vi "ReadImageParameters_JSON(SingleRack).vi"(8 "error in":errorcluster, 9 "Default JSON\nVariant in":variant, 10 "Part Name":string) -> (0 "error out":errorcluster, 2 "Error Message":string, 3 "Cam Enable-Disable Input":T1={"Top Cam"=TRUE, "Side Cam"=FALSE, "Trailing Cam"=FALSE})   [LabVIEW 2015, in "ZenGage v3.0 UI.lvclass"]
uses:
  ZenGage v3.0 UI.lvclass
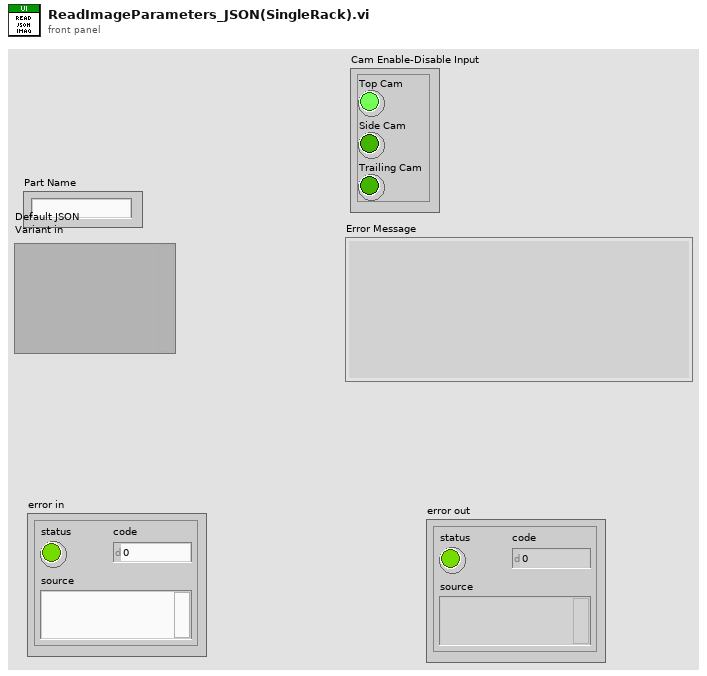
[diagram p1: front panel]
types:
  T1 = cluster{"Top Cam":bool, "Side Cam":bool, "Trailing Cam":bool}
  T2 = cluster{"CameraControllerParameters":cluster{"ID":i32, "NoOfCameras":i32, "CameraID":i32[], "NoOfReceivers":i32, "Diagnostics":cluster{"Path":string, "LightCameraSequence":cluster{"Name":string, "CameraID":i32, "LightID":i32}[], "Delaytime":i32, "DecisionParameters":cluster{"Range":i32[], "AcceptancePercentage":i32[], "Comparison":string[], "AcceptableBlackBinValue":i32}, "DiagnosticsReceiverSequence":cluster{"ReceiverName":string, "ReceiverID":i32}}, "PartsList":cluster{"Name":string, "CameraIDs":i32[], "ReceiverSequence":cluster{"ReceiverName":string, "ReceiverID":i32, "NoOfActiveCameras":i32}[]}[]}[]}
  T3 = cluster{"ID":i32, "NoOfCameras":i32, "CameraID":i32[], "NoOfReceivers":i32, "Diagnostics":cluster{"Path":string, "LightCameraSequence":cluster{"Name":string, "CameraID":i32, "LightID":i32}[], "Delaytime":i32, "DecisionParameters":cluster{"Range":i32[], "AcceptancePercentage":i32[], "Comparison":string[], "AcceptableBlackBinValue":i32}, "DiagnosticsReceiverSequence":cluster{"ReceiverName":string, "ReceiverID":i32}}, "PartsList":cluster{"Name":string, "CameraIDs":i32[], "ReceiverSequence":cluster{"ReceiverName":string, "ReceiverID":i32, "NoOfActiveCameras":i32}[]}[]}[]
  T4 = cluster{"ID":i32, "NoOfCameras":i32, "CameraID":i32[], "NoOfReceivers":i32, "Diagnostics":cluster{"Path":string, "LightCameraSequence":cluster{"Name":string, "CameraID":i32, "LightID":i32}[], "Delaytime":i32, "DecisionParameters":cluster{"Range":i32[], "AcceptancePercentage":i32[], "Comparison":string[], "AcceptableBlackBinValue":i32}, "DiagnosticsReceiverSequence":cluster{"ReceiverName":string, "ReceiverID":i32}}, "PartsList":cluster{"Name":string, "CameraIDs":i32[], "ReceiverSequence":cluster{"ReceiverName":string, "ReceiverID":i32, "NoOfActiveCameras":i32}[]}[]}
  T5 = cluster{"Name":string, "CameraIDs":i32[], "ReceiverSequence":cluster{"ReceiverName":string, "ReceiverID":i32, "NoOfActiveCameras":i32}[]}[]
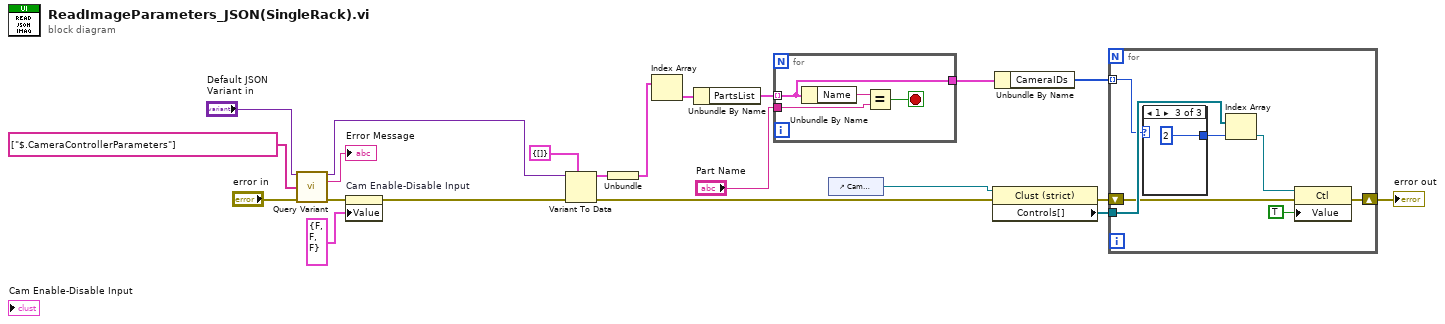
[diagram p0: block diagram]
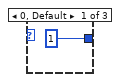
[diagram p2: hidden frame]
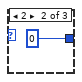
[diagram p3: hidden frame]
diagram:
  n1 = call <vilib>:"Query Variant.vi"("VCluster in"="Default JSON\nVariant in", "pathList"=string[] ["$.CameraControllerParameters"], "error IO"="error in") -> ("VCluster\n out"=w21:variant, "Error Message"=→"Error Message":string, "error out"=w2:errorcluster)  [unwired: 9 in, 1 out]
  n2 = property on="Cam Enable-Disable Input" class="Clust (strict)"(error in=w2, "Value"=T1 {"Top Cam"=FALSE, "Side Cam"=FALSE, "Trailing Cam"=FALSE} ("Cam Enable-Disable Input")) -> (error out=w1:errorcluster)  [unwired: 1 in, 1 out]
  n3 = Variant To Data(error in=w1, type=T2 {"CameraControllerParameters"=[]}, Variant=w21) -> (data=w10:T2, error out=w3:errorcluster)
  n4 = Unbundle(w10) -> ("CameraControllerParameters"=w9:T3)
  n5 = Index Array(array=w9) -> (element=w8:T4)  [unwired: 1 in]
  n6 = Unbundle By Name(w8) -> ("PartsList"=w7:T5)
  n7 = for {
    tunnel: w7 -> [w22] mode=indexing
    tunnel: "Part Name" -> [w24]
    tunnel: [w22] -> w17
    stop <- w23 stop-if-true
    n8 = Unbundle By Name(w22) -> ("Name"=w25:string)
    n9 = Equal?(x=w25, y=w24) -> (x = y?=w23:bool)
  }
  n10 = control-ref of="Cam Enable-Disable Input"() -> (w16:refnum<vi>)
  n11 = property on="Property Node" class="Clust (strict)"(reference=w16, error in=w3) -> (error out=w13:errorcluster, "Controls[]"=w14:refnum<vi>[])  [unwired: 1 out]
  n12 = Unbundle By Name(w17) -> ("CameraIDs"=w15:i32[])
  n13 = for {
    tunnel: w15 -> [w27] mode=indexing
    tunnel: w14 -> [w32]
    shift-right: [w28] -> w12
    shift-left: w13 -> [w29]
    n14 = case shown="1" w27 {
      tunnel: [1 0 2] -> w26
      frame 0, Default {
      }
      frame 2 {
      }
      frame 1 {
      }
    }
    n15 = Index Array(array=w32, index=w26) -> (element=w31:refnum<vi>)
    n16 = property class="Ctl"(reference=w31, error in=w29, "Value"=TRUE) -> (error out=w28:errorcluster)  [unwired: 1 out]
  }
  "error out" <- w12
